vi "Telnet_Write.vi"(8 "error in (no error)":errorcluster, 10 "Write Telnet Command":string, 11 "Telnet address ref":refnum<k5>) -> (0 "error out":errorcluster, 3 "connection ID out":refnum<k5>)   [LabVIEW 2018]
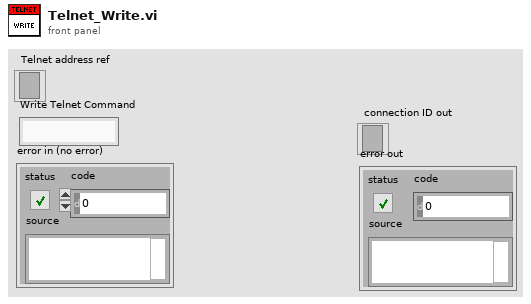
[diagram p1: front panel]
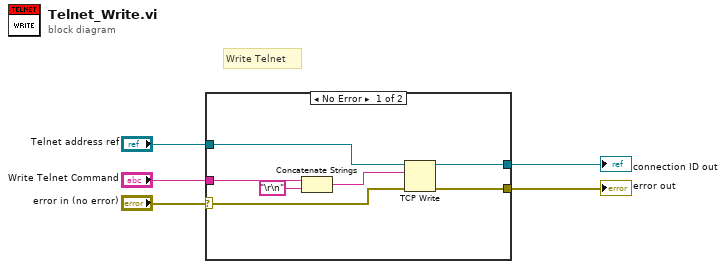
[diagram p0: block diagram]
diagram:
  # "Write Telnet"
  n1 = case shown="No Error" "error in (no error)" {
    selector: "error in (no error)" -> [w6 w14]
    tunnel: "Telnet address ref" -> [w12 w13]
    tunnel: "Write Telnet Command" -> [w10 _]
    tunnel: [w9 w13] -> w3
    tunnel: [w8 w14] -> w2
    frame No Error {
      n2 = Concatenate Strings(w10, "\r\n") -> (w11:string)
      n3 = TCP Write(connection ID=w12, data in=w11, error in (no error)=w6) -> (connection ID out=w9:refnum<k5>, error out=w8:errorcluster)  [unwired: 1 in, 1 out]
    }
    frame Error {
    }
  }
  "connection ID out" <- w3
  "error out" <- w2
